vi "create completed tour report (detailed).vi"(1 "tour number":u64, 2 "completed_tour":T1) -> (0 "completed tour (log paragraph)":string)   [LabVIEW 2020, in "main.lvlib"]
doc: "Converts the knight tour to a paragraph of text to be logged to file."
uses:
  main.lvlib
  core/core_data/completed_tour.ctl
  core/core_data/chessboard_index.ctl
  core/core_data/tour type (enum).ctl
  core/core_data/core_data.lvlib
  PTRL/string/string.lvlib
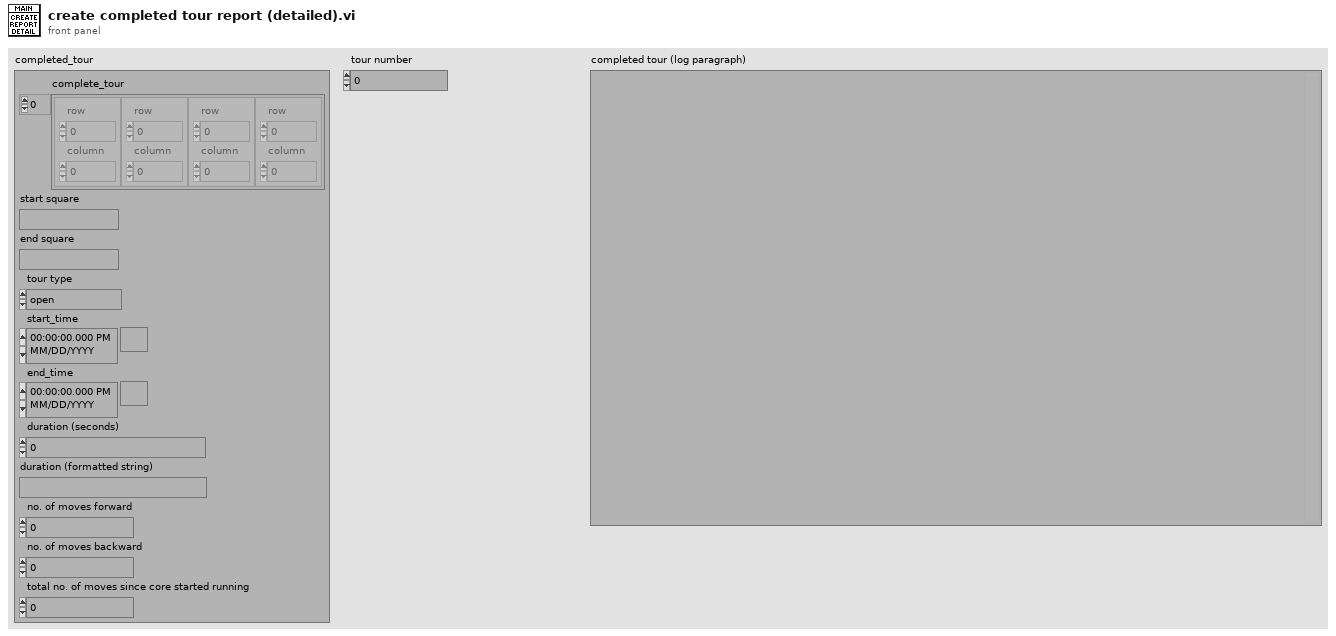
[diagram p1: front panel]
types:
  T1 = typedef "core.lvlib/core_data.lvlib/completed_tour.ctl" = cluster{"complete_tour":T2[], "start square":string, "end square":string, "tour type":T3, "start_time":timestamp, "end_time":timestamp, "duration (seconds)":dbl, "duration (formatted string)":string, "no. of moves forward":u64, "no. of moves backward":u64, "total no. of moves since core started running":u64}
  T2 = typedef "core.lvlib/core_data.lvlib/chessboard_index.ctl" = cluster{"row":u8, "column":u8}
  T3 = typedef "core.lvlib/core_data.lvlib/tour type (enum).ctl" = enum16{"open", "closed"}
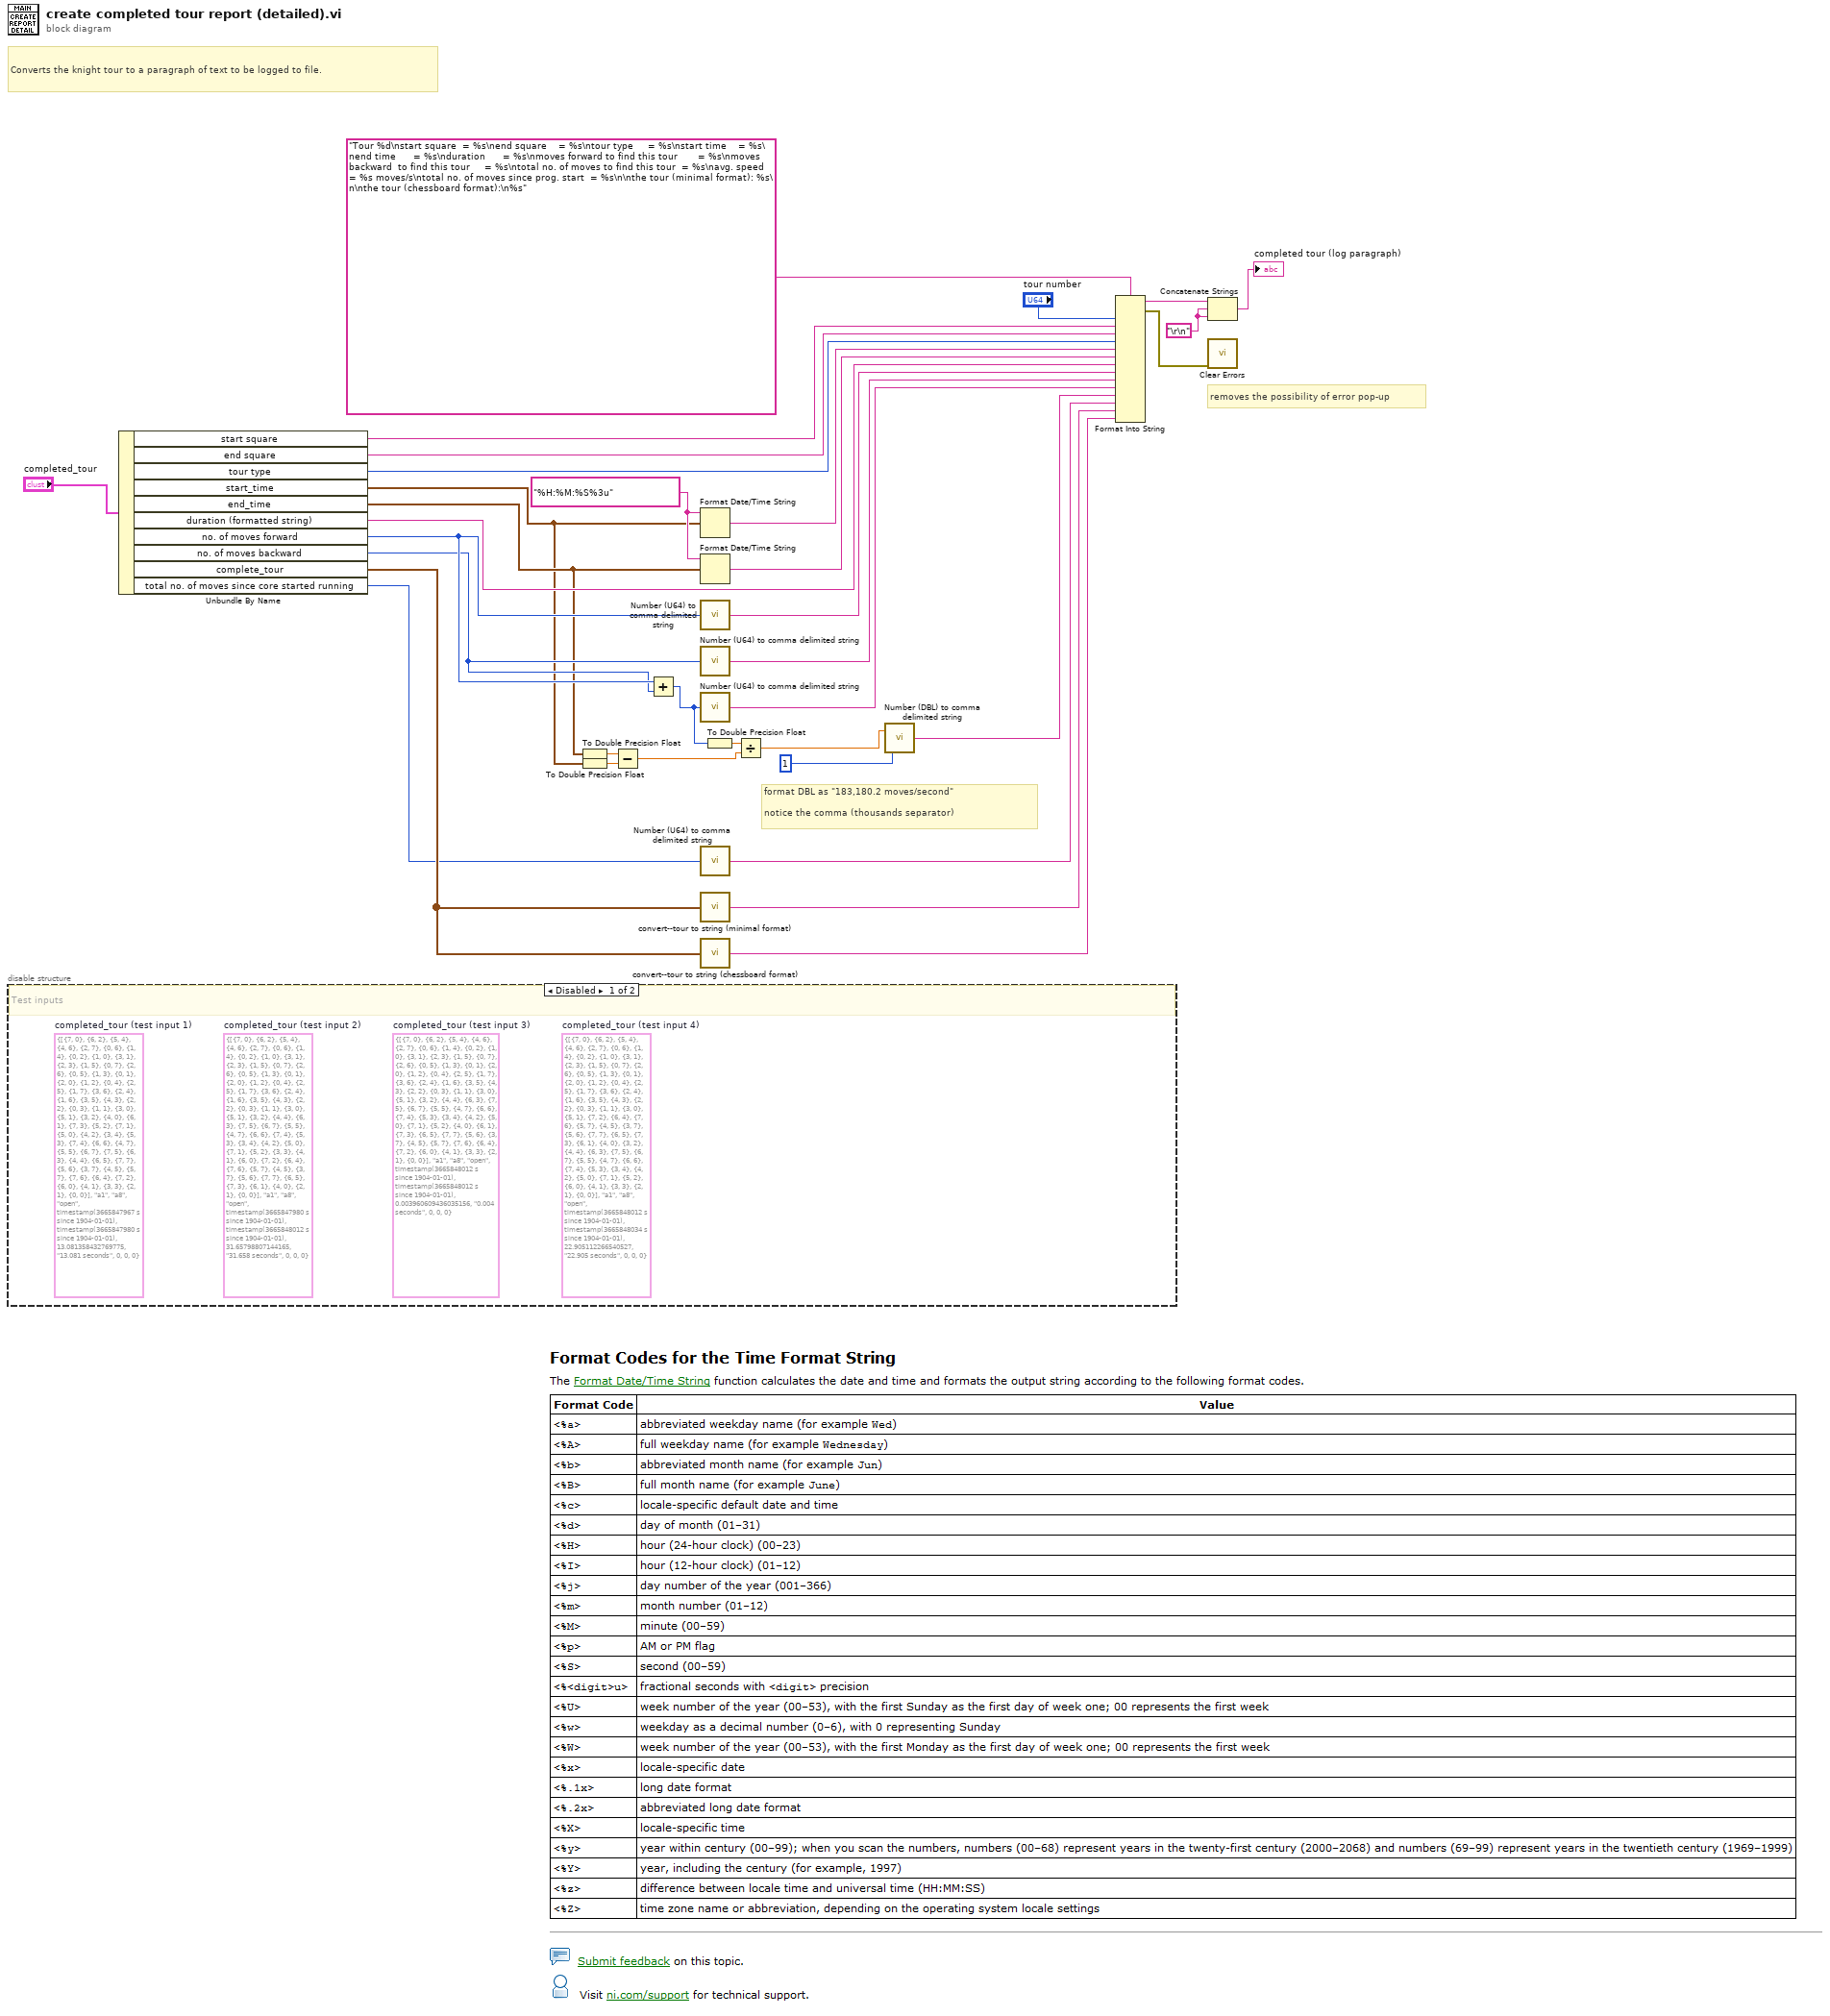
[diagram p0: block diagram]
diagram:
  w18 = "\r\n"
  w26 = "%H:%M:%S%3u" ("time format string (%c)")
  # "format DBL as \"183,180.2 moves/second\"\n\nnotice the comma (thousands separator)"
  # "removes the possibility of error pop-up"
  # "Converts the knight tour to a paragraph of text to be logged to file."
  n1 = disable-structure shown="Disabled" {
    frame Disabled {
      (unwired) T1 {"complete_tour"=[{"row"=7, "column"=0}, {"row"=6, "column"=2}, {"row"=5, "column"=4}, {"row"=4, "column"=6}, {"row"=2, "column"=7}, {"row"=0, "column"=6}, {"row"=1, "column"=4}, {"row"=0, "column"=2}, {"row"=1, "column"=0}, {"row"=3, "column"=1}, {"row"=2, "column"=3}, {"row"=1, "column"=5}, {"row"=0, "column"=7}, {"row"=2, "column"=6}, {"row"=0, "column"=5}, {"row"=1, "column"=3}, {"row"=0, "column"=1}, {"row"=2, "column"=0}, {"row"=1, "column"=2}, {"row"=0, "column"=4}, {"row"=2, "column"=5}, {"row"=1, "column"=7}, {"row"=3, "column"=6}, {"row"=2, "column"=4}, {"row"=1, "column"=6}, {"row"=3, "column"=5}, {"row"=4, "column"=3}, {"row"=2, "column"=2}, {"row"=0, "column"=3}, {"row"=1, "column"=1}, {"row"=3, "column"=0}, {"row"=5, "column"=1}, {"row"=7, "column"=2}, {"row"=6, "column"=4}, {"row"=7, "column"=6}, {"row"=5, "column"=7}, {"row"=4, "column"=5}, {"row"=3, "column"=7}, {"row"=5, "column"=6}, {"row"=7, "column"=7}, {"row"=6, "column"=5}, {"row"=7, "column"=3}, {"row"=6, "column"=1}, {"row"=4, "column"=0}, {"row"=3, "column"=2}, {"row"=4, "column"=4}, {"row"=6, "column"=3}, {"row"=7, "column"=5}, {"row"=6, "column"=7}, {"row"=5, "column"=5}, {"row"=4, "column"=7}, {"row"=6, "column"=6}, {"row"=7, "column"=4}, {"row"=5, "column"=3}, {"row"=3, "column"=4}, {"row"=4, "column"=2}, {"row"=5, "column"=0}, {"row"=7, "column"=1}, {"row"=5, "column"=2}, {"row"=6, "column"=0}, {"row"=4, "column"=1}, {"row"=3, "column"=3}, {"row"=2, "column"=1}, {"row"=0, "column"=0}], "start square"="a1", "end square"="a8", "tour type"=enum."open", "start_time"=timestamp(3665848012.019379 s since 1904-01-01), "end_time"=timestamp(3665848034.9244914 s since 1904-01-01), "duration (seconds)"=22.905112266540527, "duration (formatted string)"="22.905 seconds", "no. of moves forward"=0, "no. of moves backward"=0, "total no. of moves since core started running"=0}  # completed_tour (test input 4)
      (unwired) T1 {"complete_tour"=[{"row"=7, "column"=0}, {"row"=6, "column"=2}, {"row"=5, "column"=4}, {"row"=4, "column"=6}, {"row"=2, "column"=7}, {"row"=0, "column"=6}, {"row"=1, "column"=4}, {"row"=0, "column"=2}, {"row"=1, "column"=0}, {"row"=3, "column"=1}, {"row"=2, "column"=3}, {"row"=1, "column"=5}, {"row"=0, "column"=7}, {"row"=2, "column"=6}, {"row"=0, "column"=5}, {"row"=1, "column"=3}, {"row"=0, "column"=1}, {"row"=2, "column"=0}, {"row"=1, "column"=2}, {"row"=0, "column"=4}, {"row"=2, "column"=5}, {"row"=1, "column"=7}, {"row"=3, "column"=6}, {"row"=2, "column"=4}, {"row"=1, "column"=6}, {"row"=3, "column"=5}, {"row"=4, "column"=3}, {"row"=2, "column"=2}, {"row"=0, "column"=3}, {"row"=1, "column"=1}, {"row"=3, "column"=0}, {"row"=5, "column"=1}, {"row"=3, "column"=2}, {"row"=4, "column"=4}, {"row"=6, "column"=3}, {"row"=7, "column"=5}, {"row"=6, "column"=7}, {"row"=5, "column"=5}, {"row"=4, "column"=7}, {"row"=6, "column"=6}, {"row"=7, "column"=4}, {"row"=5, "column"=3}, {"row"=3, "column"=4}, {"row"=4, "column"=2}, {"row"=5, "column"=0}, {"row"=7, "column"=1}, {"row"=5, "column"=2}, {"row"=4, "column"=0}, {"row"=6, "column"=1}, {"row"=7, "column"=3}, {"row"=6, "column"=5}, {"row"=7, "column"=7}, {"row"=5, "column"=6}, {"row"=3, "column"=7}, {"row"=4, "column"=5}, {"row"=5, "column"=7}, {"row"=7, "column"=6}, {"row"=6, "column"=4}, {"row"=7, "column"=2}, {"row"=6, "column"=0}, {"row"=4, "column"=1}, {"row"=3, "column"=3}, {"row"=2, "column"=1}, {"row"=0, "column"=0}], "start square"="a1", "end square"="a8", "tour type"=enum."open", "start_time"=timestamp(3665848012.0154185 s since 1904-01-01), "end_time"=timestamp(3665848012.019379 s since 1904-01-01), "duration (seconds)"=0.003960609436035156, "duration (formatted string)"="0.004 seconds", "no. of moves forward"=0, "no. of moves backward"=0, "total no. of moves since core started running"=0}  # completed_tour (test input 3)
      (unwired) T1 {"complete_tour"=[{"row"=7, "column"=0}, {"row"=6, "column"=2}, {"row"=5, "column"=4}, {"row"=4, "column"=6}, {"row"=2, "column"=7}, {"row"=0, "column"=6}, {"row"=1, "column"=4}, {"row"=0, "column"=2}, {"row"=1, "column"=0}, {"row"=3, "column"=1}, {"row"=2, "column"=3}, {"row"=1, "column"=5}, {"row"=0, "column"=7}, {"row"=2, "column"=6}, {"row"=0, "column"=5}, {"row"=1, "column"=3}, {"row"=0, "column"=1}, {"row"=2, "column"=0}, {"row"=1, "column"=2}, {"row"=0, "column"=4}, {"row"=2, "column"=5}, {"row"=1, "column"=7}, {"row"=3, "column"=6}, {"row"=2, "column"=4}, {"row"=1, "column"=6}, {"row"=3, "column"=5}, {"row"=4, "column"=3}, {"row"=2, "column"=2}, {"row"=0, "column"=3}, {"row"=1, "column"=1}, {"row"=3, "column"=0}, {"row"=5, "column"=1}, {"row"=3, "column"=2}, {"row"=4, "column"=4}, {"row"=6, "column"=3}, {"row"=7, "column"=5}, {"row"=6, "column"=7}, {"row"=5, "column"=5}, {"row"=4, "column"=7}, {"row"=6, "column"=6}, {"row"=7, "column"=4}, {"row"=5, "column"=3}, {"row"=3, "column"=4}, {"row"=4, "column"=2}, {"row"=5, "column"=0}, {"row"=7, "column"=1}, {"row"=5, "column"=2}, {"row"=3, "column"=3}, {"row"=4, "column"=1}, {"row"=6, "column"=0}, {"row"=7, "column"=2}, {"row"=6, "column"=4}, {"row"=7, "column"=6}, {"row"=5, "column"=7}, {"row"=4, "column"=5}, {"row"=3, "column"=7}, {"row"=5, "column"=6}, {"row"=7, "column"=7}, {"row"=6, "column"=5}, {"row"=7, "column"=3}, {"row"=6, "column"=1}, {"row"=4, "column"=0}, {"row"=2, "column"=1}, {"row"=0, "column"=0}], "start square"="a1", "end square"="a8", "tour type"=enum."open", "start_time"=timestamp(3665847980.3574305 s since 1904-01-01), "end_time"=timestamp(3665848012.0154185 s since 1904-01-01), "duration (seconds)"=31.65798807144165, "duration (formatted string)"="31.658 seconds", "no. of moves forward"=0, "no. of moves backward"=0, "total no. of moves since core started running"=0}  # completed_tour (test input 2)
      (unwired) T1 {"complete_tour"=[{"row"=7, "column"=0}, {"row"=6, "column"=2}, {"row"=5, "column"=4}, {"row"=4, "column"=6}, {"row"=2, "column"=7}, {"row"=0, "column"=6}, {"row"=1, "column"=4}, {"row"=0, "column"=2}, {"row"=1, "column"=0}, {"row"=3, "column"=1}, {"row"=2, "column"=3}, {"row"=1, "column"=5}, {"row"=0, "column"=7}, {"row"=2, "column"=6}, {"row"=0, "column"=5}, {"row"=1, "column"=3}, {"row"=0, "column"=1}, {"row"=2, "column"=0}, {"row"=1, "column"=2}, {"row"=0, "column"=4}, {"row"=2, "column"=5}, {"row"=1, "column"=7}, {"row"=3, "column"=6}, {"row"=2, "column"=4}, {"row"=1, "column"=6}, {"row"=3, "column"=5}, {"row"=4, "column"=3}, {"row"=2, "column"=2}, {"row"=0, "column"=3}, {"row"=1, "column"=1}, {"row"=3, "column"=0}, {"row"=5, "column"=1}, {"row"=3, "column"=2}, {"row"=4, "column"=0}, {"row"=6, "column"=1}, {"row"=7, "column"=3}, {"row"=5, "column"=2}, {"row"=7, "column"=1}, {"row"=5, "column"=0}, {"row"=4, "column"=2}, {"row"=3, "column"=4}, {"row"=5, "column"=3}, {"row"=7, "column"=4}, {"row"=6, "column"=6}, {"row"=4, "column"=7}, {"row"=5, "column"=5}, {"row"=6, "column"=7}, {"row"=7, "column"=5}, {"row"=6, "column"=3}, {"row"=4, "column"=4}, {"row"=6, "column"=5}, {"row"=7, "column"=7}, {"row"=5, "column"=6}, {"row"=3, "column"=7}, {"row"=4, "column"=5}, {"row"=5, "column"=7}, {"row"=7, "column"=6}, {"row"=6, "column"=4}, {"row"=7, "column"=2}, {"row"=6, "column"=0}, {"row"=4, "column"=1}, {"row"=3, "column"=3}, {"row"=2, "column"=1}, {"row"=0, "column"=0}], "start square"="a1", "end square"="a8", "tour type"=enum."open", "start_time"=timestamp(3665847967.276072 s since 1904-01-01), "end_time"=timestamp(3665847980.3574305 s since 1904-01-01), "duration (seconds)"=13.081358432769775, "duration (formatted string)"="13.081 seconds", "no. of moves forward"=0, "no. of moves backward"=0, "total no. of moves since core started running"=0}  # completed_tour (test input 1)
      # "Test inputs"
    }
    frame Enabled {
    }
  }
  n2 = Unbundle By Name("completed_tour") -> ("start square"=w29:string, "end square"=w28:string, "tour type"=w27:T3, "start_time"=w11:timestamp, "end_time"=w12:timestamp, "duration (formatted string)"=w23:string, "no. of moves forward"=w17:u64, "no. of moves backward"=w15:u64, "complete_tour"=w21:T2[], "total no. of moves since core started running"=w2:u64)
  n3 = To Double Precision Float(number=w12) -> (double precision float=w10:dbl)
  n4 = To Double Precision Float(number=w11) -> (double precision float=w9:dbl)
  n5 = Subtract(x=w10, y=w9) -> (x-y=w6:dbl)
  n6 = Add(x=w17, y=w15) -> (x+y=w8:u64)
  n7 = Format Date/Time String(time format string (%c)=w26, seconds (now)=w11) -> (date/time string=w25:string)  [unwired: 1 in]
  n8 = Format Date/Time String(time format string (%c)=w26, seconds (now)=w12) -> (date/time string=w24:string)  [unwired: 1 in]
  n9 = call "Number (U64) to comma delimited string.vi"("Number"=w17) -> ("Comma delimited string"=w16:string)
  n10 = call "Number (U64) to comma delimited string.vi"("Number"=w15) -> ("Comma delimited string"=w14:string)
  n11 = call "Number (U64) to comma delimited string.vi"("Number"=w8) -> ("Comma delimited string"=w13:string)
  n12 = call "Number (U64) to comma delimited string.vi"("Number"=w2) -> ("Comma delimited string"=w1:string)
  n13 = call "convert--tour to string (minimal format).vi"("tour"=w21) -> ("tour (minimal format)"=w22:string)
  n14 = call "convert--tour to string (chessboard format).vi"("tour"=w21) -> ("tour (chessboard format)"=w20:string)
  n15 = To Double Precision Float(number=w8) -> (double precision float=w7:dbl)
  n16 = Divide(x=w7, y=w6) -> (x/y=w5:dbl)
  n17 = call "Number (DBL) to comma delimited string.vi"("precision (no. of decimals)"=i16 1 ("precision (6)"), "Number"=w5) -> ("Comma delimited string"=w3:string)
  n18 = Format Into String(format string="Tour %d\nstart square  = %s\nend square    = %s\ntour type     = %s\nstart time    = %s\nend time      = %s\nduration      = %s\nmoves forward to find this tour       = %s\nmoves backward  to find this tour     = %s\ntotal no. of moves to find this tour  = %s\navg. speed                            = %s moves/s\ntotal no. of moves since prog. start  = %s\n\nthe tour (minimal format): %s\n\nthe tour (chessboard format):\n%s", "tour number", w29, w28, w27, w25, w24, w23, w16, w14, w13, w3, w1, w22, w20) -> (resulting string=w33:string, error out=w31:errorcluster)  [unwired: 2 in]
  n19 = Concatenate Strings(w33, w18, w18) -> (→"completed tour (log paragraph)":string)
  n20 = call <vilib>:"Clear Errors.vi"("error in (no error)"=w31) -> ()  [unwired: 5 in, 2 out]
